vi "Get Configured Performance Channels.vi"(8 "error in (no error)":errorcluster, 11 "VeriStand Data Sharing Framework in":refnum<class "VeriStand DSF.lvclass">) -> (0 "error out":errorcluster, 2 "performance channel offsets":u64[](array[numeric]) format="%.0x", 3 "VeriStand Data Sharing Framework out":refnum<class "VeriStand DSF.lvclass">)   [LabVIEW 2017, in "DSF Engine.lvlib" / "VeriStand DSF.lvclass"]
uses:
  VeriStand DSF.lvclass
  VeriStand DSF.lvclass/VeriStand DSF.ctl
  <vilib>/NI Veristand/Custom Device API/Data Access Type.ctl
  <vilib>/NI Veristand/Custom Device API/Custom Device API.lvlib
  Shared/DSF Shared.lvlib
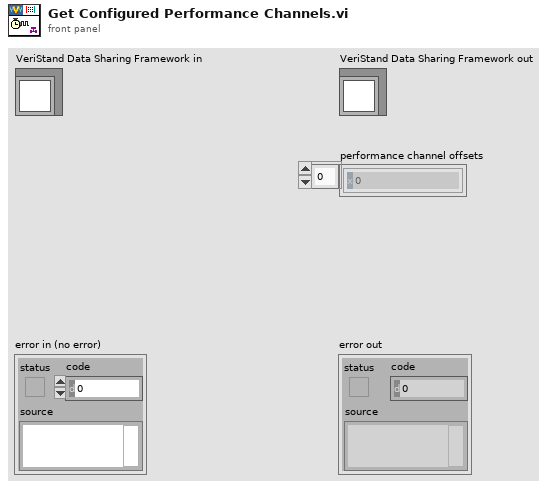
[diagram p1: front panel]
types:
  T1 = typedef "Custom Device API.lvlib/Custom Device Item Ref.ctl" = u64
  T2 = typedef "Custom Device API.lvlib/Data Access Type.ctl" = enum16{"Read", "Write"}
  T3 = typedef "Custom Device API.lvlib/Data Reference.ctl" = i32
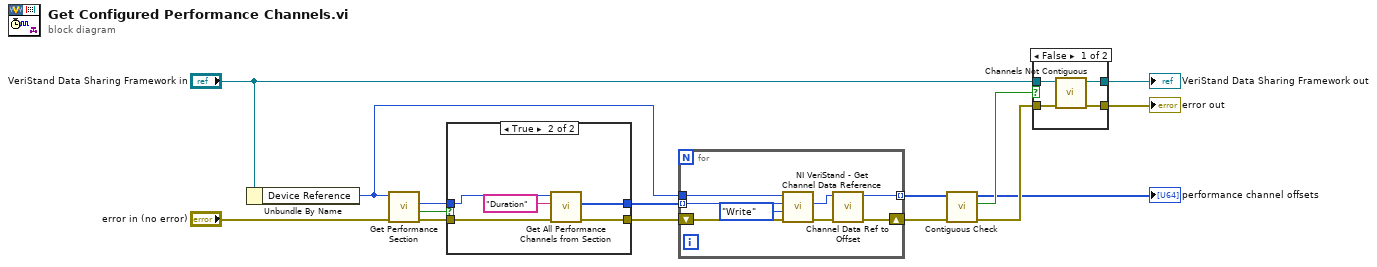
[diagram p0: block diagram]
diagram:
  n1 = Unbundle By Name("VeriStand Data Sharing Framework in") -> ("Device Reference"=w9:T1)
  n2 = call "Get Performance Section.vi"("error in (no error)"="error in (no error)", "Item Ref in"=w9) -> ("error out"=w14:errorcluster, "found"=w3:bool, "Performance Section ref"=w13:T1)  [unwired: 6 in, 1 out]
  n3 = case shown="True" w3 {
    tunnel: w14 -> [w16 w21]
    tunnel: w13 -> [_ w20]
    tunnel: [w16 w18] -> w12
    tunnel: [_ w17] -> w2
    frame False {
    }
    frame True {
      n4 = call "Get All Performance Channels from Section.vi"("error in (no error)"=w21, "Section Name"="Duration", "Item Ref in"=w20) -> ("error out"=w18:errorcluster, "performance channels refs"=w17:T1[])  [unwired: 6 in, 1 out]
    }
  }
  n5 = for {
    shift-right: [w28] -> w11
    shift-left: w12 -> [w27]
    tunnel: [w25] -> w10 mode=indexing
    tunnel: w9 -> [w23]
    tunnel: w2 -> [w22] mode=indexing
    n6 = call <vilib>:"NI VeriStand - Get Channel Data Reference.vi"("error in (no error)"=w27, "Access"=Data_Access_Type."Write", "Channel Ref in"=w22, "Device Ref in"=w23) -> ("error out"=w29:errorcluster, "Channel Data Reference"=w26:T3)  [unwired: 5 in, 1 out]
    n7 = call "Channel Data Ref to Offset.vi"("error in (no error)"=w29, "Channel Data Reference"=w26) -> ("error out"=w28:errorcluster, "channel offset"=w25:u64)  [unwired: 8 in]
  }
  n8 = call "Contiguous Check.vi"("error in (no error)"=w11, "channel offsets in"=w10) -> ("error out"=w5:errorcluster, "contiguous?"=w4:bool, "channel offsets out"=→"performance channel offsets":u64[])  [unwired: 7 in]
  n9 = case shown="False" w4 {
    tunnel: "VeriStand Data Sharing Framework in" -> [w33 w35]
    tunnel: [w32 w35] -> w7
    tunnel: [w31 w34] -> w6
    tunnel: w5 -> [w30 w34]
    frame False {
      n10 = call "Channels Not Contiguous.vi"("error in (no error)"=w30, "VeriStand DSF in"=w33) -> ("error out"=w31:errorcluster, "VeriStand DSF out"=w32:refnum<class "VeriStand DSF.lvclass">)  [unwired: 8 in]
    }
    frame True {
    }
  }
  "error out" <- w6
  "VeriStand Data Sharing Framework out" <- w7
